vi "GroupDataProtoTest.vi"() -> ()   [LabVIEW 2020, in "VectoScratch.lvlib"]
uses:
  VectoScratch.lvlib
  Vecto/proto/GroupData/Data.ctl
  Vecto/proto/GroupData/GroupData.lvlib
panel:
  out "error out":errorcluster
  out "Data":T1
  out "string":string
  in  "GroupData":T1={"group_name"="alpha", "data_timestamp"=0, "scaled_data"=[1.0, 2.0, 3.0, 4.0, 5.0], "raw_data"=[2.0, 3.0, 4.0, 5.0, 6.0]}
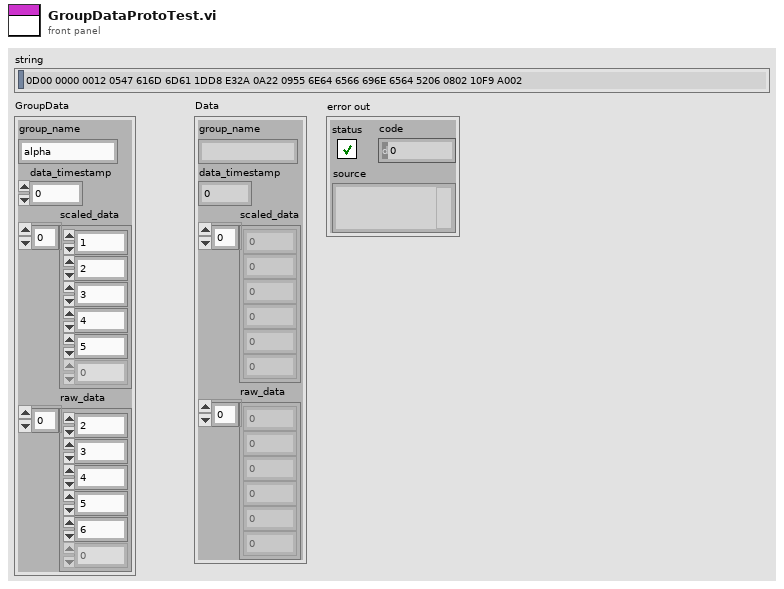
[diagram p1: front panel]
types:
  T1 = typedef "GroupData.lvlib/Data.ctl" = cluster{"group_name":string, "data_timestamp":i64, "scaled_data":dbl[], "raw_data":dbl[]}
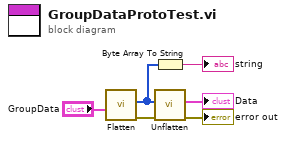
[diagram p0: block diagram]
diagram:
  n1 = call "Flatten.vi"("Data"="GroupData") -> ("error out"=w4:errorcluster, "Buffer"=w3:u8[])  [unwired: 9 in]
  n2 = Byte Array To String(unsigned byte array=w3) -> (string=→"string":string)
  n3 = call "Unflatten.vi"("error in"=w4, "Buffer"=w3) -> ("error out"=→"error out":errorcluster, "Data"=→"Data":T1)  [unwired: 8 in]
